vi "Get Module Path.vi"(8 "error in":errorcluster, 11 "Module Name":string) -> (0 "error out":errorcluster, 3 "module path":path)   [LabVIEW 2020, in "Navigation.lvlib"]
doc: "____\nHAMPEL SOFTWARE ENGINEERING v2.6.0 (2023-12-19 10:54)"
uses:
  Navigation.lvlib
  Libraries/hse-libraries/Source/hse-application/hse-application.lvclass/hse-application.ctl
  Libraries/hse-libraries/Source/hse-application/HSE Application not initialized--error.vi
  <vilib>/Utility/error.llb/Clear Errors.vi
  Libraries/hse-libraries/Source/hse-application/hse-application__GetSingleton.vi
  <vilib>/Utility/sysdir.llb/Get System Directory.vi
  <vilib>/Utility/error.llb/Error Cluster From Error Code.vi
  Libraries/hse-libraries/Source/hse-application/hse-application.lvclass
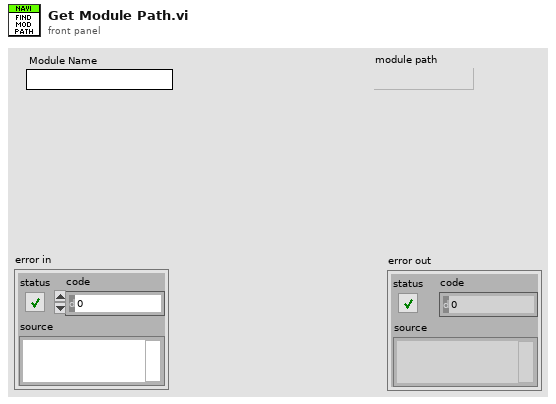
[diagram p1: front panel]
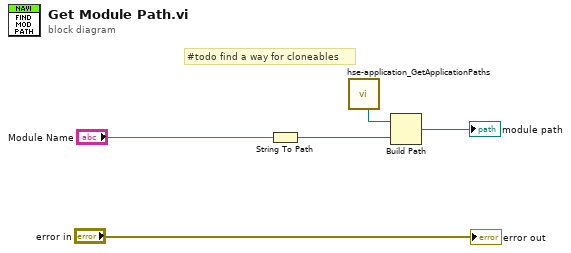
[diagram p0: block diagram]
diagram:
  # "#todo find a way for cloneables"
  n1 = String To Path(string="Module Name") -> (path=w1:path)
  n2 = call "hse-application_GetApplicationPaths.vi"() -> ("Application Base Path"=w3:path)  [unwired: 5 in, 6 out]
  n3 = Build Path(base path=w3, name or relative path=w1) -> (appended path=→"module path":path)
  "error out" <- "error in"
